vi "Launch Series.vi"(6 "Series CFG":string, 8 "error in":errorcluster, 9 "Virt Instrs":string, 10 "Instr CFGs":string[](array[string]), 11 "Study Actor in":refnum<class "Study Actor.lvclass">) -> (0 "error out":errorcluster, 3 "Study Actor out":refnum<class "Study Actor.lvclass">)   [LabVIEW 2023, in "Study Actor.lvlib" / "Study Actor.lvclass"]
uses:
  Study Actor.lvclass
  Series/Series Base/Series Base.lvclass
  Series/Series Actor/Series Actor/Series Actor.lvclass
  Study Actor.lvclass/Study Actor.ctl
  Series/Series Actor/Series Actor/Series Actor.lvclass/Series Actor.ctl
  ac49a4a7-b07b-43cf-9404-ee9b245844b6.vi
  <vilib>/JDP Science/JSONtext/Find Item.vi
  <vilib>/JDP Science/JSONtext/Next JSON Value.vi
  <vilib>/JDP Science/JSONtext/String Subset.vi
  <vilib>/JDP Science/JSONtext/Parsing/Advance past next JSON Value (inlined COPY).vi
  <vilib>/JDP Science/JSONtext/Parsing/Advance past whitespace.vi
  <vilib>/JDP Science/JSONtext/Parsing/Advance past String.vi
  <vilib>/JDP Science/JSONtext/Parsing/Advance past Number.vi
  <vilib>/JDP Science/JSONtext/Parsing/Advance past Line Ending.vi
  <vilib>/MGI/Panel Manager/Panel/Panel/Subpanel/Subpanel.lvclass
  <vilib>/JDP Science/JSONtext/Parsing/Parse Full Path or Item Name.vi
  <vilib>/JDP Science/JSONtext/Parsing/Advance past Array.vi
  <vilib>/JDP Science/JSONtext/Parsing/Advance past Object.vi
  <vilib>/JDP Science/JSONtext/support/Error Cluster From Code.vi
  <vilib>/JDP Science/JSONtext/Offset/Find Item Locations by Path.vi
  <vilib>/JDP Science/JSONtext/JSON text to Variant.vi
  <vilib>/JDP Science/JSONtext/LVClass Serializer/JSONtext LVClass Serializer.lvclass
  <vilib>/MGI/Panel Manager/Panel/Panel/Subpanel/Subpanel.vi
  <vilib>/MGI/Panel Manager/Panel Actor/Panel Actor/Panel Actor.lvclass
  <vilib>/MGI/Panel Manager/Panel/Panel.lvlib
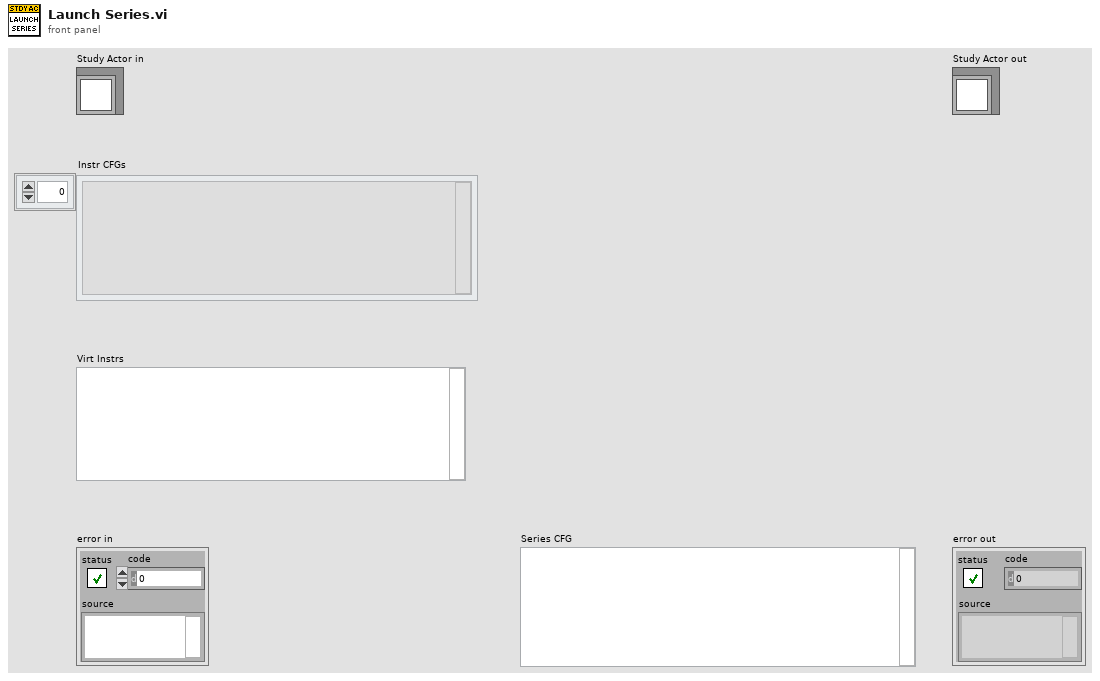
[diagram p1: front panel]
types:
  T1 = map{string, refnum<class "Message Enqueuer.lvclass">}
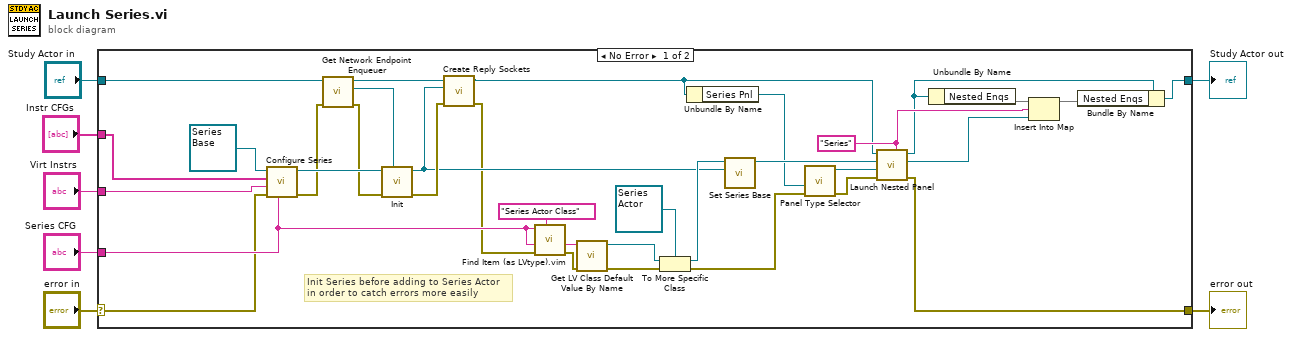
[diagram p0: block diagram]
diagram:
  n1 = case shown="No Error" "error in" {
    selector: "error in" -> [w30 w43]
    tunnel: [w24 w43] -> w6
    tunnel: [w22 w42] -> w4
    tunnel: "Study Actor in" -> [w17 w42]
    tunnel: "Series CFG" -> [w31 _]
    tunnel: "Instr CFGs" -> [w29 _]
    tunnel: "Virt Instrs" -> [w28 _]
    frame No Error {
      w26 = "Series" ("Debug Alias")
      # "Init Series before adding to Series Actor\nin order to catch errors more easily"
      n2 = call "Configure Series.vi"("Series CFG"=w31, "error in (no error)"=w30, "Virt Instrs CFG"=w28, "Instr CFGs"=w29, "HAL GOOP4:Series Base in"=refnum<class "Series Base.lvclass"> refnum ("HAL GOOP4.lvlib:Study Base.lvclass")) -> ("error out"=w16:errorcluster, "HAL GOOP4:Series Base out"=w39:refnum<class "Series Base.lvclass">)  [unwired: 5 in]
      n3 = call "Get Network Endpoint Enqueuer.vi"("error in"=w16, "Study Actor in"=w17) -> ("error out"=w15:errorcluster, "Network Endpoint Enqueuer"=w14:refnum<class "Message Enqueuer.lvclass">, "Study Actor out"=w13:refnum<class "Study Actor.lvclass">)  [unwired: 6 in, 1 out]
      n4 = call-dynamic "Init.vi"("Target Enqueuer"=w14, "error in"=w15, "HAL GOOP4:Series Base in"=w39) -> ("error out"=w12:errorcluster, "HAL GOOP4:Series Base out"=w10:refnum<class "Series Base.lvclass">)  [unwired: 7 in]
      n5 = call "Create Reply Sockets.vi"("error in"=w12, "Series Base in"=w10, "Study Actor in"=w13) -> ("error out"=w9:errorcluster, "Study Actor out"=w11:refnum<class "Study Actor.lvclass">)  [unwired: 7 in]
      n6 = call "Find Item (as LVtype).vim"("$Path or Item Name"="Series Actor Class", "error in (no error)"=w9, "Data Type and Default Value"=w31, "JSON"=w31) -> ("error out"=w34:errorcluster, "Data"=w35:string)  [unwired: 4 in, 2 out]
      n7 = call <vilib>:"Get LV Class Default Value By Name.vi"("error in (no error)"=w34, "class name"=w35) -> ("error out"=w38:errorcluster, "object"=w37:refnum<class>)  [unwired: 8 in]
      n8 = To More Specific Class(target class=refnum<class "Series Actor.lvclass"> refnum ("Series Actor.lvlib:Series Actor.lvclass"), reference=w37, error in=w38) -> (specific class reference=w32:refnum<class "Series Actor.lvclass">, error out=w8:errorcluster)
      n9 = Unbundle By Name(w11) -> ("Series Pnl"=w19:refnum<vi>)
      n10 = call "Set Series Base.vi"("Series Base"=w10, "Series Actor in"=w32) -> ("Series Actor out"=w41:refnum<class "Series Actor.lvclass">)  [unwired: 9 in]
      n11 = call-poly <vilib>:"Panel Type Selector.vi"("Error In"=w8, "Sub Panel"=w19) -> ("Error Out"=w20:errorcluster, "Subpanel Out"=w18:refnum<class "Subpanel.lvclass">)  [unwired: 8 in]
      n12 = call <vilib>:"Launch Nested Panel.vi"("Debug Alias"=w26, "error in (no error)"=w20, "Panel"=w18, "Nested Panel Actor"=w41, "Panel Actor in"=w11) -> ("error out"=w24:errorcluster, "Nested Actor's Enqueuer"=w25:refnum<class "Message Enqueuer.lvclass">, "Panel Actor out"=w23:refnum<class "Study Actor.lvclass">)  [unwired: 3 in, 1 out]
      n13 = Unbundle By Name(w23) -> ("Nested Enqs"=w27:T1)
      n14 = Insert Into Map(map in=w27, key=w26, value=w25) -> (map out=w21:T1)  [unwired: 2 out]
      n15 = Bundle By Name(cluster=w23, "Nested Enqs"=w21) -> (w22:refnum<class "Study Actor.lvclass">)
    }
    frame Error {
    }
  }
  "error out" <- w6
  "Study Actor out" <- w4
